vi "RemoveChildFromNode.vi"(8 "error in":errorcluster, 10 "removed child":T1, 11 "Engine Parent Editor Node in":refnum<class "Engine Parent Editor Node.lvclass">) -> (0 "error out":errorcluster, 3 "Engine Parent Editor Node out":refnum<class "Engine Parent Editor Node.lvclass">)   [LabVIEW 2013, in "PL Framework Configuration Tool.lvlib" / "Engine Parent Editor Node.lvclass"]
uses:
  Engine Parent Editor Node.lvclass
  <vilib>/NI/Configuration Framework/Node/NodeRef.ctl
  <vilib>/NI/Configuration Framework/Node/NISE_CEF_Node.lvclass
  <vilib>/NI/Configuration Framework/serializable node/NISE_CEF_serializable node.lvclass
  <vilib>/NI/Configuration Framework/serializable configuration/NISE_CEF_serializable configuration.lvclass/NISE_CEF_serializable configuration.ctl
  <vilib>/NI/Module Execution Interface/Engine Configuration/engine configuration.lvclass
  TBM Configuration Node/TBM Configuration Node.lvclass
  <vilib>/Utility/LVClass/Get LV Class Name.vi
  <vilib>/NI/Configuration Framework/error generator/NISE_error generator.vi
  read engine configuration.vi
  write engine configuration.vi
  <vilib>/NI/Configuration Framework/serializable configuration/NISE_CEF_serializable configuration.lvclass
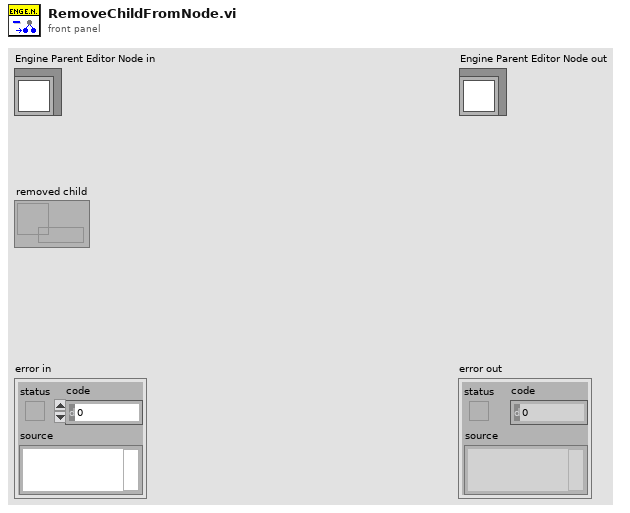
[diagram p1: front panel]
types:
  T1 = typedef "NISE_CEF_Node.lvclass/NodeRef.ctl" = refnum<data-value>
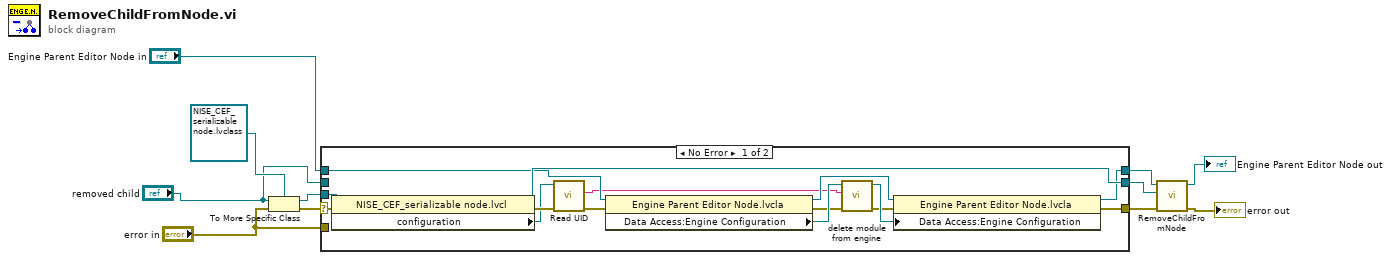
[diagram p0: block diagram]
diagram:
  n1 = To More Specific Class(target class=refnum<data-value> refnum, reference="removed child", error in="error in") -> (specific class reference=w10:refnum<data-value>, error out=w8:errorcluster)
  n2 = case shown="No Error" w8 {
    selector: w8 -> [w23 _]
    tunnel: [w17 w29] -> w7
    tunnel: [w25 w28] -> w11
    tunnel: w10 -> [w24 _]
    tunnel: "error in" -> [_ w29]
    tunnel: "removed child" -> [_ w28]
    tunnel: "Engine Parent Editor Node in" -> [w21 w27]
    tunnel: [w19 w27] -> w6
    frame No Error {
      n3 = property class="NISE_CEF_serializable node.lvcl"(reference=w24, error in=w23) -> (reference out=w25:refnum<data-value>, error out=w26:errorcluster, "configuration"=w22:refnum<class "NISE_CEF_serializable configuration.lvclass">)
      n4 = call <vilib>:"Read UID.vi"("error in"=w26, "configuration in"=w22) -> ("error out"=w20:errorcluster, "instance id"=w12:string)  [unwired: 7 in, 1 out]
      n5 = property class="Engine Parent Editor Node.lvcla"(reference=w21, error in=w20) -> (reference out=w18:refnum<class "Engine Parent Editor Node.lvclass">, error out=w13:errorcluster, "Data Access:Engine Configuration"=w16:refnum<class "engine configuration.lvclass">)
      n6 = call-dynamic "delete module from engine.vi"("error in"=w13, "module ID"=w12, "engine configuration in"=w16) -> ("error out"=w14:errorcluster, "engine configuration out"=w15:refnum<class "engine configuration.lvclass">)  [unwired: 7 in]
      n7 = property class="Engine Parent Editor Node.lvcla"(reference=w18, error in=w14, "Data Access:Engine Configuration"=w15) -> (reference out=w19:refnum<class "Engine Parent Editor Node.lvclass">, error out=w17:errorcluster)
    }
    frame Error {
    }
  }
  n8 = call-parent "RemoveChildFromNode.vi"("error in"=w7, "removed child"=w11, "NISE_CEF_Node in"=w6) -> ("error out"=→"error out":errorcluster, "NISE_CEF_Node out"=→"Engine Parent Editor Node out":refnum<class "Engine Parent Editor Node.lvclass">)  [unwired: 7 in]
